vi "Read Period.vi"(8 "error in (no error)":errorcluster, 11 "Framework Performance in":refnum<class "Performance.lvclass">) -> (0 "error out":errorcluster, 2 "period":u32 format="%d us", 3 "Framework Performance out":refnum<class "Performance.lvclass">)   [LabVIEW 2019, in "DSF Core.lvlib" / "Performance.lvclass"]
uses:
  Performance.lvclass
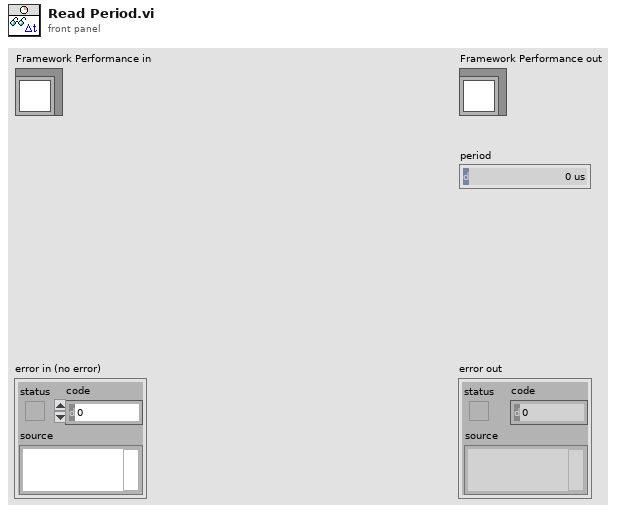
[diagram p1: front panel]
types:
  T1 = typedef "DSF Core.lvlib/Timing Status Pointer.lvclass/Timing Status Data.ctl" = cluster{"rx start time":u32, "rx end time":u32, "tx start time":u32, "tx end time":u32, "cycle start time":u32, "cycle end time":u32, "prev start time":u32}
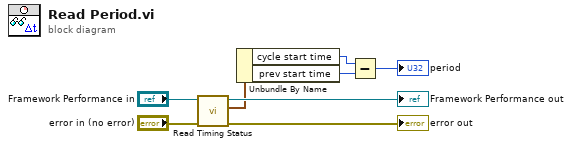
[diagram p0: block diagram]
diagram:
  n1 = call "Read Timing Status.vi"("error in (no error)"="error in (no error)", "Framework Performance in"="Framework Performance in") -> ("error out"=→"error out":errorcluster, "timing status"=w4:T1, "Framework Performance out"=→"Framework Performance out":refnum<class "Performance.lvclass">)  [unwired: 7 in]
  n2 = Unbundle By Name(w4) -> ("cycle start time"=w3:u32, "prev start time"=w2:u32)
  n3 = Subtract(x=w3, y=w2) -> (x-y=→"period":u32)
